vi "mod_Extract SSB pilot tone.vi"(0 "passband waveform":waveform(dbl), 5 "pilot extraction filter":T2={"taps"=81, "approx freq. (Hz)"=0.0, "search (+/- % of Fsampl) "=0.25}, 11 "error in (no error)":errorcluster, 13 "reset? (T)":bool=TRUE) -> (4 "extracted AM modulated wfm (IF)":waveform(dbl), 6 "extracted pilot tone wfm (IF)":waveform(dbl), 8 "filter information":T1 {"Pilot rejection filter"."df" format="%.2p"; "Pilot rejection filter"."f0" format="%.2p"; "Pilot rejection filter"."Mag H(w)" format="%.2p"; "Pilot extraction filter"."df" format="%.2p"; "Pilot extraction filter"."f0" format="%.2p"; "Pilot extraction filter"."Mag H(w)" format="%.2p"}, 15 "error out":errorcluster)   [LabVIEW 2020, in "niAMT.lvlib"]
uses:
  <vilib>/addons/Modulation/niAMT.lvlib
  <vilib>/addons/Modulation/Analog/controls/mod_AM pilot extraction filter.ctl
  <vilib>/addons/Modulation/Analog/controls/mod_AM pilot filter info.ctl
  <vilib>/Analysis/3filter.llb/IIR Filter (DBL).vi
  <vilib>/Analysis/NI_AALBase.lvlib
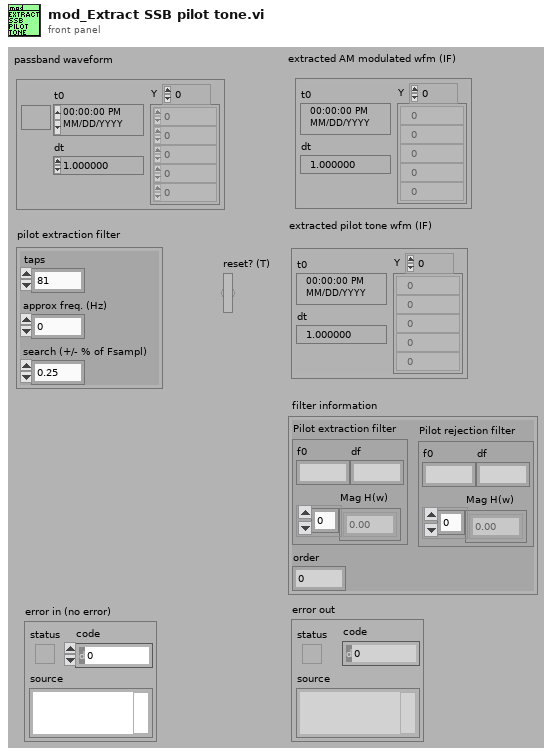
[diagram p1: front panel]
types:
  T1 = typedef "niAMT.lvlib/mod_AM pilot filter info.ctl" = cluster{"Pilot extraction filter":cluster{"f0":dbl, "df":dbl, "Mag H(w)":dbl[]}, "order":i32, "Pilot rejection filter":cluster{"f0":dbl, "df":dbl, "Mag H(w)":dbl[]}}
  T2 = typedef "niAMT.lvlib/mod_AM pilot extraction filter.ctl" = cluster{"taps":i32, "approx freq. (Hz)":dbl, "search (+/- % of Fsampl) ":dbl}
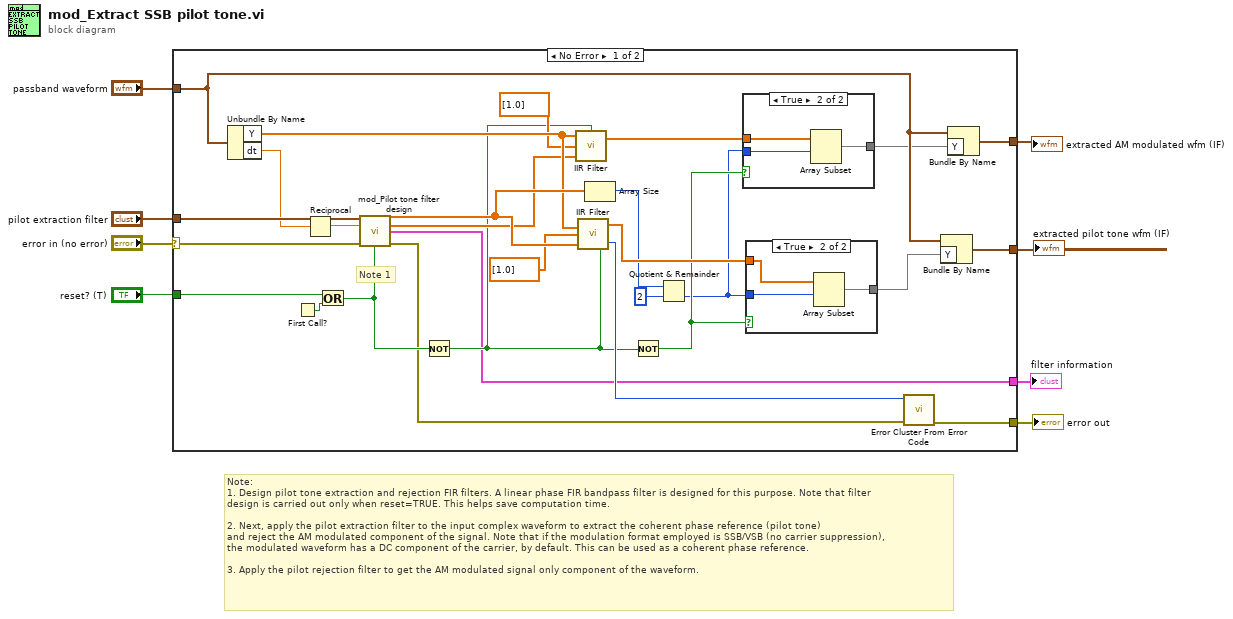
[diagram p0: block diagram]
diagram:
  # "Note:\n1. Design pilot tone extraction and rejection FIR filters. A linear phase FIR bandpass filter is designed for this purpose. Note that filter\ndesign is carried out only when reset=TRUE. This helps save computation time.\n\n2. Next, apply the pilot extraction filter to the input complex waveform to extract the coherent phase reference (pilot tone)\nand reject the AM modulated component of the signal. Note that if the modulation format employed is SSB/VSB (no carrier suppression), \nthe modulated waveform has a DC component of the carrier, by default. This can be used as a coherent phase reference.\n\n3. Apply the pilot rejection filter to get the AM modulated signal only component of the waveform."
  n1 = case shown="No Error" "error in (no error)" {
    selector: "error in (no error)" -> [w31 w45]
    tunnel: [w26 _] -> w5
    tunnel: [w25 _] -> w7
    tunnel: [w28 w45] -> w6
    tunnel: "passband waveform" -> [w27 _]
    tunnel: "pilot extraction filter" -> [w15 _]
    tunnel: "reset? (T)" -> [w35 _]
    tunnel: [w12 _] -> w1
    frame No Error {
      # "Note 1"
      n2 = Unbundle By Name(w27) -> ("Y"=w23:dbl[], "dt"=w14:dbl)
      n3 = First Call?() -> (First Call?: T/F=w36:bool)
      n4 = Reciprocal(x=w14) -> (1/x=w13:dbl)
      n5 = Or(x=w35, y=w36) -> (x .or. y?=w34:bool)
      n6 = call <vilib>:"mod_Pilot tone filter design.vi"("pilot extraction filter"=w15, "sampling frequency"=w13, "error in (no error)"=w31, "reset? (T)"=w34) -> ("pilot extraction filter coefficients"=w32:dbl[], "pilot rejection filter coefficients"=w21:dbl[], "filter information"=w12:T1, "error out"=w30:errorcluster)  [unwired: 8 out]
      n7 = Not(x=w34) -> (.not. x?=w20:bool)
      n8 = call-poly <vilib>:"IIR Filter.vi"("init/cont (init:F)"=w20, "Forward Coefficients"=w21, "Reverse Coefficients"=dbl[] [1.0], "X"=w23) -> ("Filtered X"=w19:dbl[])  [unwired: 1 out]
      n9 = call-poly <vilib>:"IIR Filter.vi"("init/cont (init:F)"=w20, "Forward Coefficients"=w32, "Reverse Coefficients"=dbl[] [1.0], "X"=w23) -> ("error"=w29:i32, "Filtered X"=w33:dbl[])
      n10 = Array Size(array=w32) -> (size(s)=w10:i32)
      n11 = Not(x=w20) -> (.not. x?=w18:bool)
      n12 = Quotient & Remainder(x=w10, y=2) -> (floor(x/y)=w11:i32)  [unwired: 1 out]
      n13 = case shown="True" w18 {
        tunnel: w19 -> [w37 w40]
        tunnel: [w37 w39] -> w17
        tunnel: w11 -> [_ w38]
        frame False {
        }
        frame True {
          n14 = Array Subset(array=w40, index=w38) -> (w39:dbl[])  [unwired: 1 in]
        }
      }
      n15 = case shown="True" w18 {
        tunnel: w33 -> [w41 w44]
        tunnel: [w41 w43] -> w24
        tunnel: w11 -> [_ w42]
        frame False {
        }
        frame True {
          n16 = Array Subset(array=w44, index=w42) -> (w43:dbl[])  [unwired: 1 in]
        }
      }
      n17 = call <vilib>:"Error Cluster From Error Code.vi"("error in (no error)"=w30, "error code (0)"=w29) -> ("error out"=w28:errorcluster)  [unwired: 1 in, 6 out]
      n18 = Bundle By Name(cluster=w27, "Y"=w24) -> (w25:waveform(dbl))
      n19 = Bundle By Name(cluster=w27, "Y"=w17) -> (w26:waveform(dbl))
    }
    frame Error {
    }
  }
  "error out" <- w6
  "extracted pilot tone wfm (IF)" <- w7
  "extracted AM modulated wfm (IF)" <- w5
  "filter information" <- w1
